vi "TDMS to Meta Data.vi"(6 "Channel name":string, 7 "Group name":string, 8 "Error In":errorcluster, 9 "Name":string, 10 "Value":variant, 11 "tdms file":refnum<k34>) -> (0 "Error Out":errorcluster, 1 "found?":bool, 2 "Variant out":variant, 3 "tdms file out":refnum<k34>)   [LabVIEW 2016]
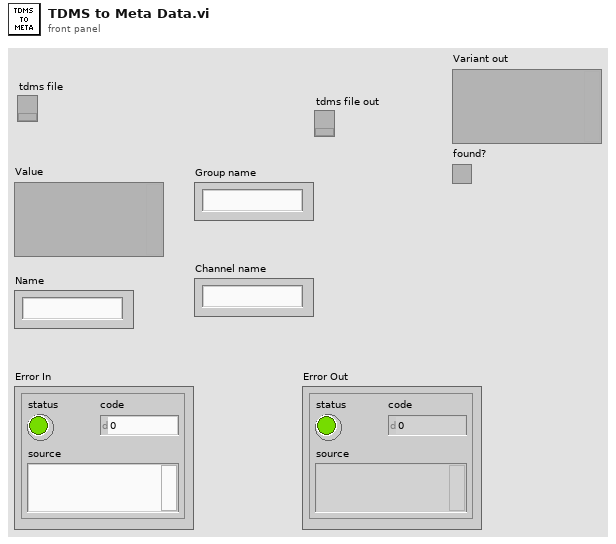
[diagram p1: front panel]
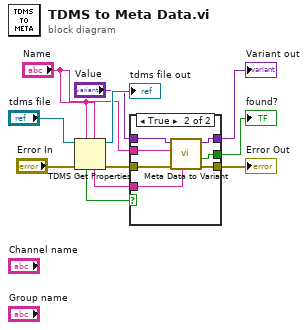
[diagram p0: block diagram]
diagram:
  n1 = TDMS Get Properties(5:"Name", 7:"Name", 8:"Error In", 11:"tdms file") -> (0:w4:errorcluster, 3:→"tdms file out":refnum<k34>, 4:w8:string, 6:w9:bool)  [unwired: 2 in, 2 out]
  n2 = case shown="True" w9 {
    tunnel: w8 -> [_ w20]
    tunnel: "Value" -> [w13 w19]
    tunnel: [w13 w18] -> w6
    tunnel: [_ w17] -> w5
    tunnel: w4 -> [w12 w16]
    tunnel: [w12 w15] -> w2
    tunnel: "Name" -> [_ w14]
    frame False {
    }
    frame True {
      n3 = call "Meta Data to Variant.vi"("Meta data"=w20, "Error In"=w16, "Section"=w14, "Value"=w19) -> ("Error Out"=w15:errorcluster, "found?"=w17:bool, "Variant out"=w18:variant)  [unwired: 4 in, 1 out]
    }
  }
  "Error Out" <- w2
  "Variant out" <- w6
  "found?" <- w5
